vi "Inttcp.vi"(1 "String":string) -> (0 "TCP Network Connection Refnum":refnum<k5>)   [LabVIEW 2014]
panel:
  out "data out":string
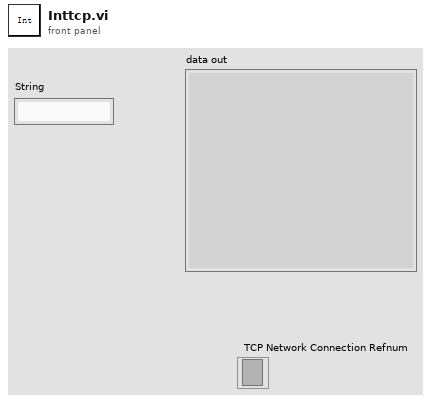
[diagram p1: front panel]
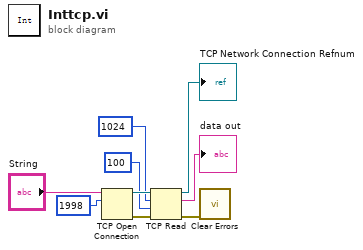
[diagram p0: block diagram]
diagram:
  n1 = TCP Open Connection(address="String", remote port or service name=u16 1998) -> (connection ID=w8:refnum<k5>, error out=w1:errorcluster)  [unwired: 3 in]
  n2 = TCP Read(connection ID=w8, bytes to read=1024, error in (no error)=w1, 9:100 ("timeout ms (25000)")) -> (connection ID out=→"TCP Network Connection Refnum":refnum<k5>, data out=→"data out":string, error out=w4:errorcluster)  [unwired: 1 in]
  n3 = call <vilib>:"Clear Errors.vi"("error in (no error)"=w4) -> ()  [unwired: 5 in, 2 out]
